vi "_Parse IEM I32 Result.vi"(8 "error in (no error)":errorcluster, 10 "Input String":string, 11 "VISA resource name":refnum<visa-resource-name>) -> (0 "error out":errorcluster, 1 "Results":T1 {"Out Of Tolerance" format="%^.3e"}, 2 "Reliability":i32, 3 "VISA resource name out":refnum<visa-resource-name>)   [LabVIEW 2020, in "Rohde&Schwarz CMXP NR FR2 Measurement.lvlib"]
uses:
  <instrlib>/Rohde&Schwarz CMXP NR FR2 Measurement/Rohde&Schwarz CMXP NR FR2 Measurement.lvlib
  <instrlib>/Rohde&Schwarz CMXP NR FR2 Measurement/Private/rsidr_core.llb/rsidr_core.lvlib
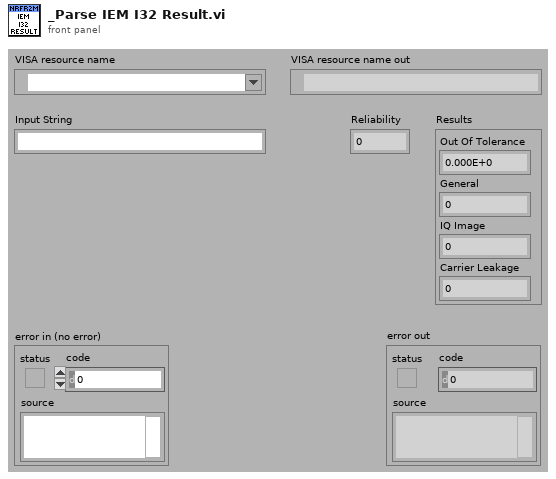
[diagram p1: front panel]
types:
  T1 = cluster{"Out Of Tolerance":dbl, "General":i32, "IQ Image":i32, "Carrier Leakage":i32}
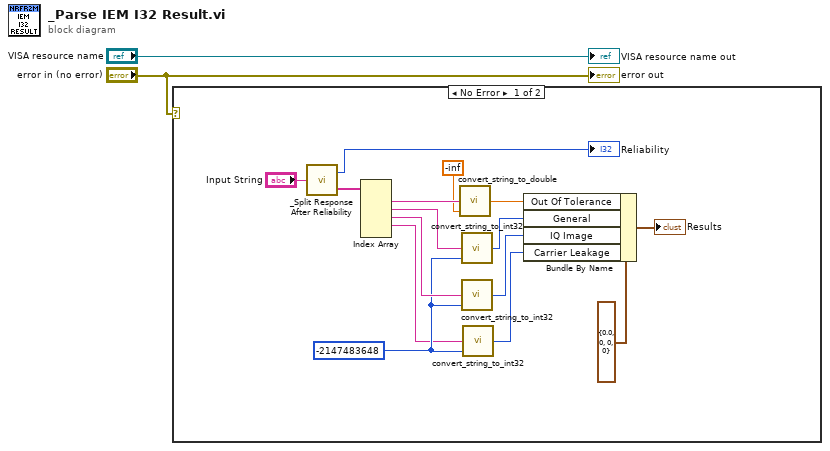
[diagram p0: block diagram]
diagram:
  n1 = case shown="No Error" "error in (no error)" {
    frame No Error {
      w8 = -2147483648
      n2 = call <instrlib>:"_Split Response After Reliability.vi"("Input String"="Input String") -> ("Response out"=w12:string[], "Reliability out"=→"Reliability":i32)
      n3 = Index Array(array=w12) -> (element #1=w11:string, element #2=w10:string, element #3=w9:string, element #4=w7:string)  [unwired: 5 in, 1 out]
      n4 = call <instrlib>:"convert_string_to_double.vi"("default (0)"=-inf, "String in"=w11) -> ("double value out"=w17:dbl)  [unwired: 3 in]
      n5 = call <instrlib>:"convert_string_to_int32.vi"("default (0)"=w8, "String in"=w10) -> ("int32 value out"=w16:i32)  [unwired: 3 in]
      n6 = call <instrlib>:"convert_string_to_int32.vi"("default (0)"=w8, "String in"=w9) -> ("int32 value out"=w15:i32)  [unwired: 3 in]
      n7 = call <instrlib>:"convert_string_to_int32.vi"("default (0)"=w8, "String in"=w7) -> ("int32 value out"=w5:i32)  [unwired: 3 in]
      n8 = Bundle By Name(cluster=T1 {"Out Of Tolerance"=0.0, "General"=0, "IQ Image"=0, "Carrier Leakage"=0} ("Results"), "Out Of Tolerance"=w17, "General"=w16, "IQ Image"=w15, "Carrier Leakage"=w5) -> (→"Results":T1)
    }
    frame Error {
    }
  }
  "VISA resource name out" <- "VISA resource name"
  "error out" <- "error in (no error)"
